vi "Check Connection Error.vi"(8 "error in (no error)":errorcluster, 11 "TCP_Streamer_Subscriber in":refnum<class "TCP_Streamer_Subscriber.lvclass">) -> (0 "error out":errorcluster, 3 "TCP_Streamer_Subscriber out":refnum<class "TCP_Streamer_Subscriber.lvclass">)   [LabVIEW 2021, in "TCP_Streamer_Subscriber.lvclass"]
uses:
  TCP_Streamer_Subscriber.lvclass
  TCP_Streamer_Subscriber.lvclass/TCP_Streamer_Subscriber.ctl
  Typedef/State.ctl
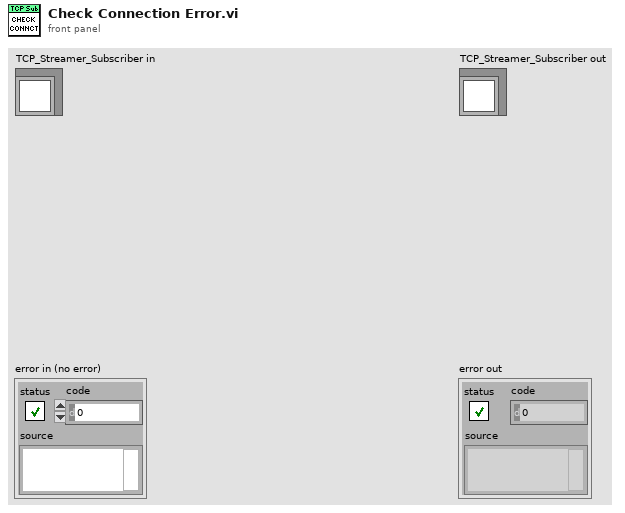
[diagram p1: front panel]
types:
  T1 = typedef "TCP_Streamer_Subscriber.lvclass/State.ctl" = enum16{"Stopped", "Connecting", "Receiving"}
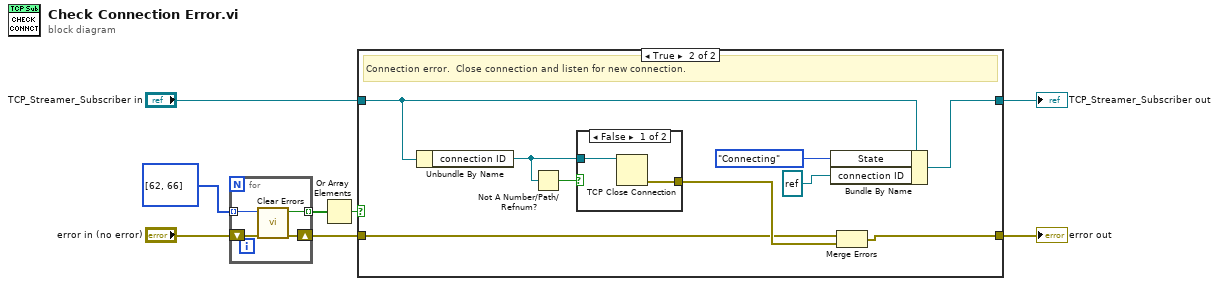
[diagram p0: block diagram]
diagram:
  n1 = for {
    tunnel: [w11] -> w6 mode=indexing
    shift-right: [w10] -> w8
    shift-left: "error in (no error)" -> [w12]
    tunnel: i32[] [62, 66] -> [w9] mode=indexing
    n2 = call <vilib>:"Clear Errors.vi"("error in (no error)"=w12, "specific error code to clear (0: all)"=w9) -> ("error out"=w10:errorcluster, "specific error cleared?"=w11:bool)  [unwired: 4 in]
  }
  n3 = Or Array Elements(Boolean array=w6) -> (logical OR=w5:bool)
  n4 = case shown="True" w5 {
    tunnel: "TCP_Streamer_Subscriber in" -> [w14 w21]
    tunnel: w8 -> [w13 w18]
    tunnel: [w14 w16] -> w2
    tunnel: [w13 w17] -> w1
    frame False {
    }
    frame True {
      # "Connection error.  Close connection and listen for new connection."
      n5 = Unbundle By Name(w21) -> ("connection ID"=w19:refnum<k5>)
      n6 = Not A Number/Path/Refnum?(number/path/refnum=w19) -> (NaN/Path/Refnum?=w20:bool)
      n7 = case shown="False" w20 {
        tunnel: [w25 _] -> w22
        tunnel: w19 -> [w24 _]
        frame False {
          n8 = TCP Close Connection(connection ID=w24) -> (error out=w25:errorcluster)  [unwired: 2 in, 1 out]
        }
        frame True {
        }
      }
      n9 = Bundle By Name(cluster=w21, "State"=State."Connecting", "connection ID"=refnum<k5> refnum) -> (w16:refnum<class "TCP_Streamer_Subscriber.lvclass">)
      n10 = Merge Errors(w18, w22) -> (w17:errorcluster)
    }
  }
  "error out" <- w1
  "TCP_Streamer_Subscriber out" <- w2
